vi "GOOP_ClassSettingsMemory.vi"(0 "Library Refnum":refnum<vi>, 1 "Action":T3, 2 "LvClassIconSettingsIn":T2 {"Frame thickness" min=1 max=3 step=1}, 3 "ItemIconIn":string, 5 "error in":errorcluster) -> (14 "Library Refnum":refnum<vi>, 15 "Found":bool, 16 "LvClassIconSettings":T2 {"Frame thickness" min=1 max=3 step=1}, 17 "ItemIcon":string, 18 "Type":T1, 19 "error out":errorcluster)   [LabVIEW 2020]
uses:
  <resource>/Framework/Providers/Open_GDS/ClassProviders/Common/LvClass_class/GDSLvClass_IconSettingsType.ctl
  <resource>/Framework/Providers/Open_GDS/SubVIs/GOOP_ClassSettingsMemory_Action.ctl
  <resource>/Framework/Providers/Open_GDS/ClassProviders/Common/LvIcon_class/GDSLvIcon_Type.ctl
  <resource>/Framework/Providers/Open_GDS/ClassProviders/Common/LvClass_class/GDSLvClass_IconSettingsNames.ctl
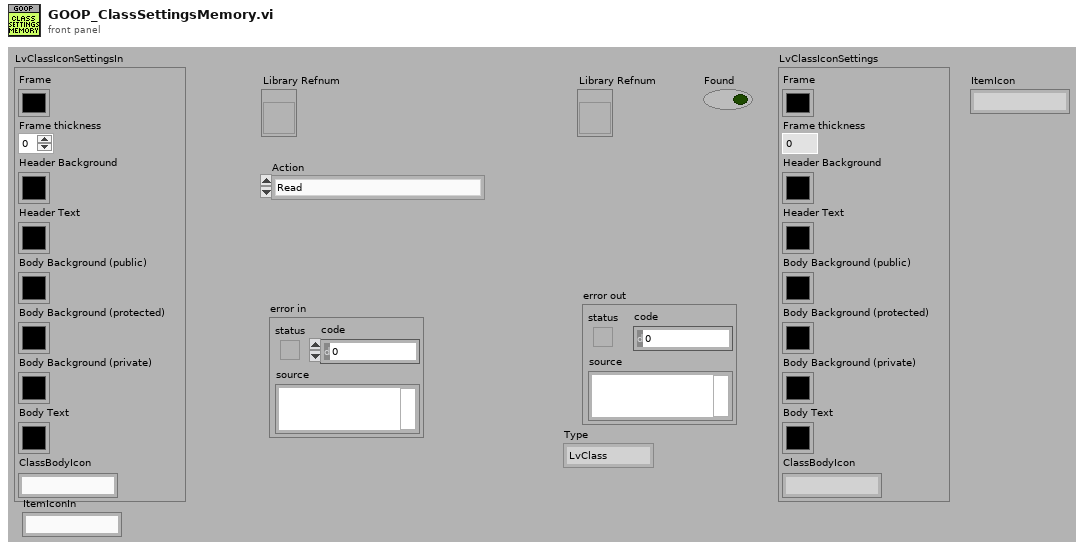
[diagram p1: front panel]
types:
  T1 = typedef "GDSLvIcon_Type.ctl" = enum16{"LvClass", "Library", "X-Control", "LvInterface"}
  T2 = typedef "GDSLvClass_IconSettingsType.ctl" = cluster{"Frame":u32, "Frame thickness":u8, "Header Background":u32, "Header Text":u32, "ColorPublic":u32, "ColorProtected":u32, "ColorPrivate":u32, "Body Text":u32, "ClassBodyIcon":string}
  T3 = typedef "GOOP_ClassSettingsMemory_Action.ctl" = enum16{"Read", "Write", "Read (ClassItemIconOnly)"}
  T4 = typedef "GDSLvClass_IconSettingsNames.ctl" = enum16{"EndevoGOOP_ColorFrame", "EndevoGOOP_FrameThickness", "EndevoGOOP_ColorHeader", "EndevoGOOP_ColorTextHeader", "EndevoGOOP_ColorPublic", "EndevoGOOP_ColorProtected", "EndevoGOOP_ColorPrivate", "EndevoGOOP_ColorTextBody", "EndevoGOOP_ClassItemIcon", "EndevoGOOP_ClassBodyIcon"}
  T5 = cluster{"LvClassIconSettingsIn":T2, "ItemIconIn":string}
  T6 = cluster{"LvClassIconSettings":T2, "ItemIcon":string}
  T7 = cluster{"LvClassIconSettings":T2, "ItemIcon":string}[]
  T8 = cluster{"LvClassIconSettingsIn":T2, "ItemIconIn":string}[]
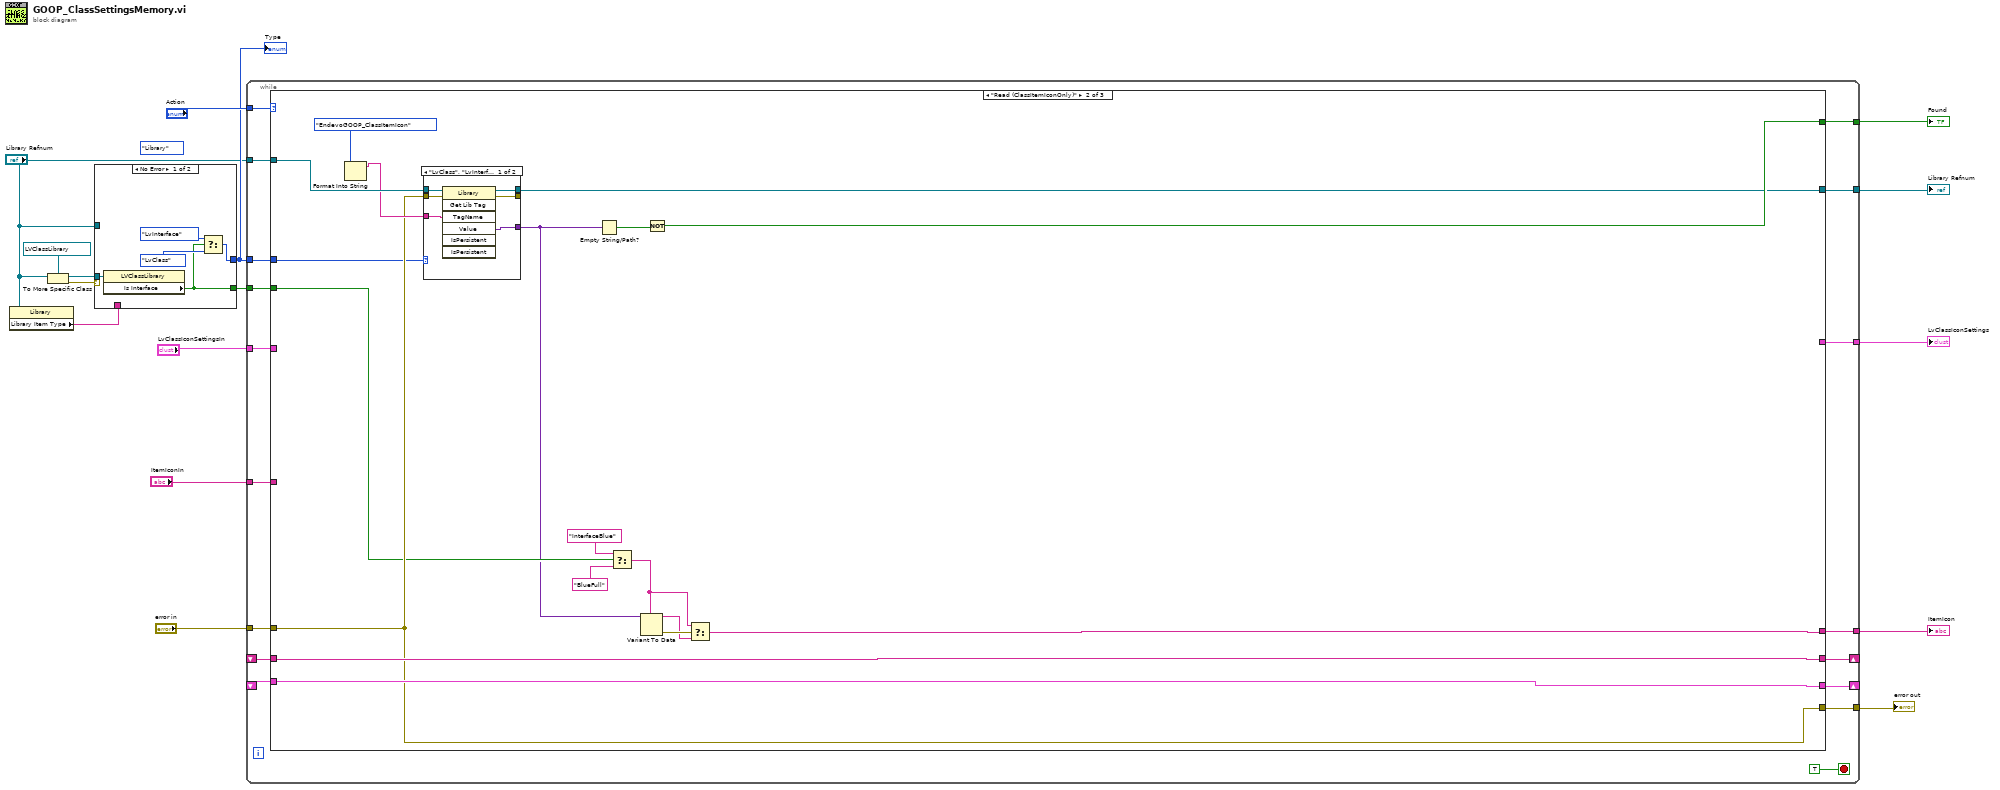
[diagram p0: block diagram]
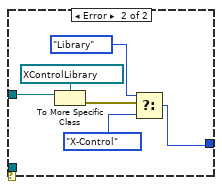
[diagram p2: hidden frame]
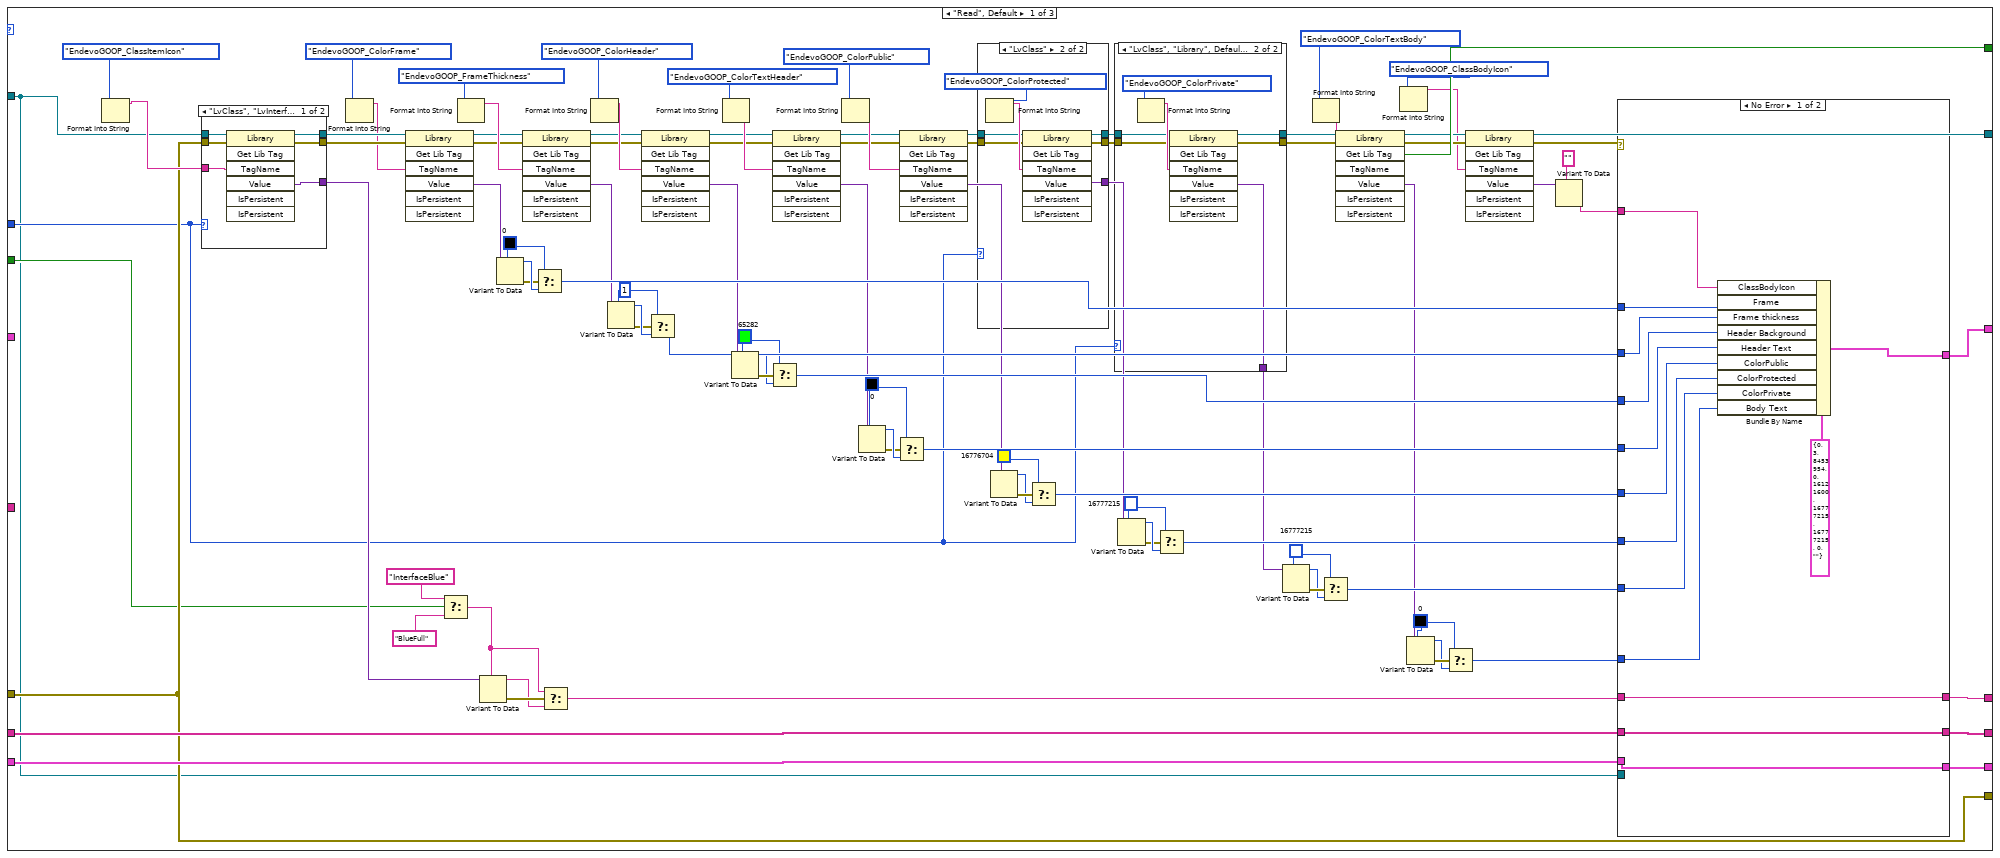
[diagram p3: hidden frame]
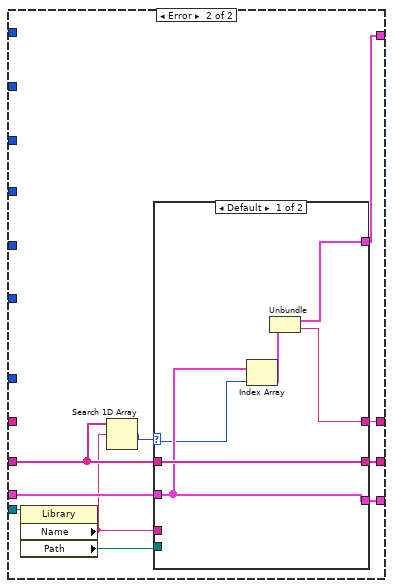
[diagram p7: hidden frame]
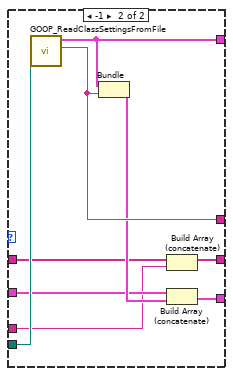
[diagram p8: hidden frame]
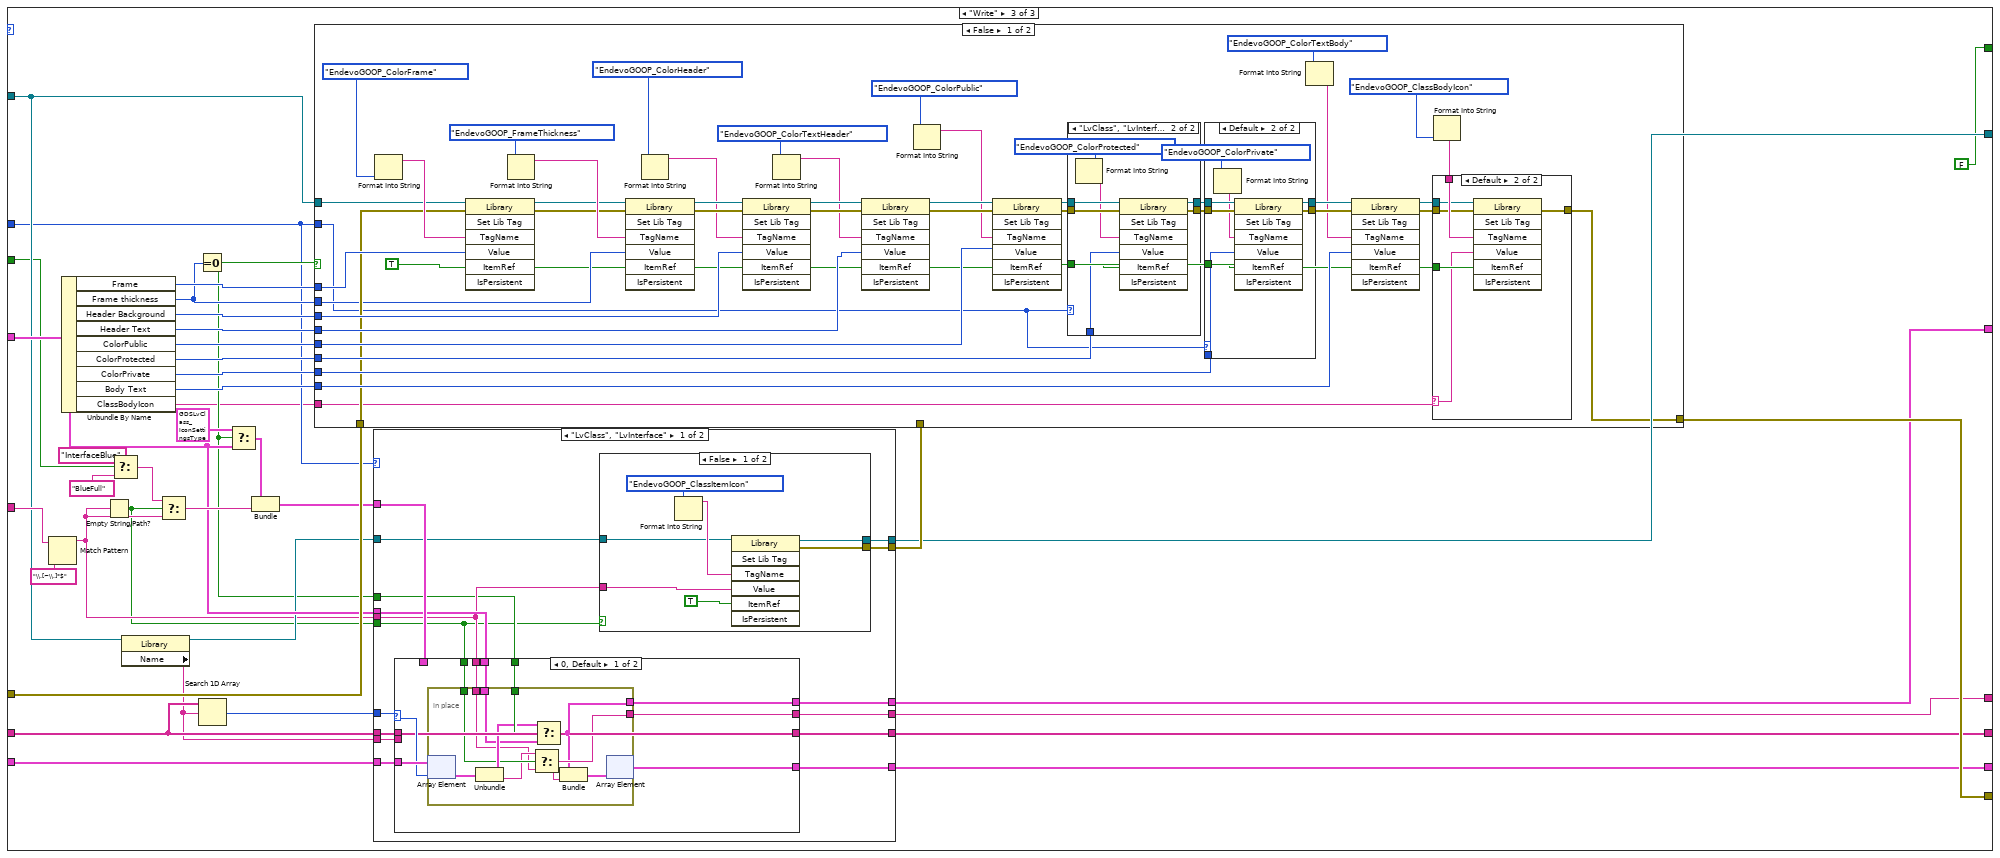
[diagram p10: hidden frame]
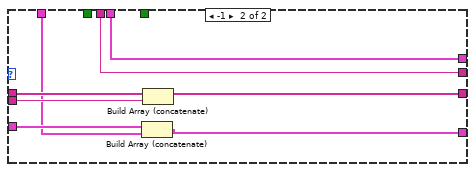
[diagram p12: hidden frame]
diagram:
  (unwired) GDSLvIcon_Type."Library" ("Type")
  n1 = property class="Library"(reference="Library Refnum") -> ("Library Item Type"=w3:string)  [unwired: 1 in, 2 out]
  n2 = To More Specific Class(target class=refnum<vi> refnum ("reference"), reference="Library Refnum") -> (specific class reference=w2:refnum<vi>, error out=w5:errorcluster)  [unwired: 1 in]
  n3 = case shown="No Error" w5 {
    tunnel: "Library Refnum" -> [_ w26]
    tunnel: [w18 w24] -> w6
    tunnel: w3 -> [_ _]
    tunnel: w2 -> [w21 _]
    tunnel: [w17 _] -> w1
    frame No Error {
      n4 = property class="LVClassLibrary"(reference=w21) -> ("Is Interface"=w17:bool)  [unwired: 1 in, 2 out]
      n5 = Select(t=GDSLvIcon_Type."LvInterface" ("Type"), s=w17, f=GDSLvIcon_Type."LvClass" ("Type")) -> (s? t:f=w18:T1)
    }
    frame Error {
      n6 = To More Specific Class(target class=refnum<vi> refnum ("reference"), reference=w26) -> (error out=w25:errorcluster)  [unwired: 1 in, 1 out]
      n7 = Select(t=GDSLvIcon_Type."Library" ("Type"), s=w25, f=GDSLvIcon_Type."X-Control" ("Type")) -> (s? t:f=w24:T1)
    }
  }
  "Type" <- w6
  n8 = while {
    tunnel: [w44] -> w16
    tunnel: [w43] -> w15
    tunnel: "Library Refnum" -> [w42]
    tunnel: "error in" -> [w41]
    tunnel: [w40] -> w13
    tunnel: [w39] -> w12
    shift-right: [w36] -> _
    shift-left: _ -> [w37]
    shift-right: [w35] -> _
    shift-left: _ -> [w34]
    tunnel: "Action" -> [w33]
    tunnel: "LvClassIconSettingsIn" -> [w32]
    tunnel: [w31] -> w9
    tunnel: "ItemIconIn" -> [w30]
    tunnel: w6 -> [w29]
    tunnel: w1 -> [w28]
    stop <- TRUE stop-if-true
    n9 = case shown="\"Read (ClassItemIconOnly)\"" w33 {
      tunnel: [w141 w224 w249] -> w44
      tunnel: [w140 _ w250] -> w43
      tunnel: w42 -> [w45 w222 w239]
      tunnel: w41 -> [w60 w216 w264]
      tunnel: [w101 w208 FALSE ("GetTag")] -> w40
      tunnel: [w55 w207 w242] -> w39
      tunnel: w37 -> [w64 w218 w261]
      tunnel: [w63 w218 w251] -> w36
      tunnel: [w62 w217 w252] -> w35
      tunnel: w34 -> [w61 w217 w255]
      tunnel: w32 -> [_ _ w253]
      tunnel: [w60 w216 w259] -> w31
      tunnel: w30 -> [_ _ w246]
      tunnel: w29 -> [w59 w215 w238]
      tunnel: w28 -> [w49 w214 w236]
      frame "Read", Default {
        w106 = u32 16777215 ("Frame")
        w97 = u32 0 ("Frame")
        w95 = u32 16777215 ("Frame")
        w89 = u32 16776704 ("Frame")
        w87 = u32 0 ("Frame")
        w81 = u32 65282 ("Frame")
        w79 = u8 1 ("Frame thickness")
        w77 = u32 0 ("Frame")
        n10 = Format Into String(GDSLvClass_IconSettingsNames."EndevoGOOP_ClassItemIcon" ("Enum")) -> (resulting string=w127:string)  [unwired: 3 in, 1 out]
        n11 = case shown="\"LvClass\", \"LvInterface\"" w59 {
          tunnel: [w165 _] -> w129
          tunnel: w45 -> [w164 w167]
          tunnel: w127 -> [w163 _]
          tunnel: [w162 w166] -> w126
          tunnel: [w161 w167] -> w125
          tunnel: w60 -> [w160 w166]
          frame "LvClass", "LvInterface" {
            n12 = invoke class="Library" method="Get Lib Tag"(reference=w164, error in=w160, "TagName"=w163) -> (reference out=w161:refnum<vi>, error out=w162:errorcluster, "Value"=w165:variant)  [unwired: 4 in, 4 out]
          }
          frame Default {
          }
        }
        n13 = Format Into String(GDSLvClass_IconSettingsNames."EndevoGOOP_ColorFrame" ("Enum")) -> (resulting string=w111:string)  [unwired: 3 in, 1 out]
        n14 = invoke class="Library" method="Get Lib Tag"(reference=w125, error in=w126, "TagName"=w111) -> (reference out=w65:refnum<vi>, error out=w112:errorcluster, "Value"=w71:variant)  [unwired: 4 in, 4 out]
        n15 = Select(t="InterfaceBlue", s=w49, f="BlueFull") -> (s? t:f=w46:string)
        n16 = Format Into String(GDSLvClass_IconSettingsNames."EndevoGOOP_FrameThickness" ("Enum")) -> (resulting string=w113:string)  [unwired: 3 in, 1 out]
        n17 = Variant To Data(type=w46, Variant=w129) -> (data=w128:string, error out=w130:errorcluster)  [unwired: 1 in]
        n18 = Variant To Data(type=w77, Variant=w71) -> (data=w76:u32, error out=w75:errorcluster)  [unwired: 1 in]
        n19 = invoke class="Library" method="Get Lib Tag"(reference=w65, error in=w112, "TagName"=w113) -> (reference out=w68:refnum<vi>, error out=w114:errorcluster, "Value"=w72:variant)  [unwired: 4 in, 4 out]
        n20 = Select(t=w77, s=w75, f=w76) -> (s? t:f=w131:u32)
        n21 = Select(t=w46, s=w130, f=w128) -> (s? t:f=w139:string)
        n22 = Format Into String(GDSLvClass_IconSettingsNames."EndevoGOOP_ColorHeader" ("Enum")) -> (resulting string=w115:string)  [unwired: 3 in, 1 out]
        n23 = Variant To Data(type=w79, Variant=w72) -> (data=w80:u8, error out=w78:errorcluster)  [unwired: 1 in]
        n24 = invoke class="Library" method="Get Lib Tag"(reference=w68, error in=w114, "TagName"=w115) -> (reference out=w66:refnum<vi>, error out=w67:errorcluster, "Value"=w84:variant)  [unwired: 4 in, 4 out]
        n25 = Select(t=w79, s=w78, f=w80) -> (s? t:f=w132:u8)
        n26 = Format Into String(GDSLvClass_IconSettingsNames."EndevoGOOP_ColorTextHeader" ("Enum")) -> (resulting string=w116:string)  [unwired: 3 in, 1 out]
        n27 = Variant To Data(type=w81, Variant=w84) -> (data=w82:u32, error out=w83:errorcluster)  [unwired: 1 in]
        n28 = Select(t=w81, s=w83, f=w82) -> (s? t:f=w133:u32)
        n29 = invoke class="Library" method="Get Lib Tag"(reference=w66, error in=w67, "TagName"=w116) -> (reference out=w69:refnum<vi>, error out=w70:errorcluster, "Value"=w88:variant)  [unwired: 4 in, 4 out]
        n30 = Format Into String(GDSLvClass_IconSettingsNames."EndevoGOOP_ColorPublic" ("Enum")) -> (resulting string=w117:string)  [unwired: 3 in, 1 out]
        n31 = Variant To Data(type=w87, Variant=w88) -> (data=w86:u32, error out=w85:errorcluster)  [unwired: 1 in]
        n32 = Select(t=w87, s=w85, f=w86) -> (s? t:f=w134:u32)
        n33 = invoke class="Library" method="Get Lib Tag"(reference=w69, error in=w70, "TagName"=w117) -> (reference out=w73:refnum<vi>, error out=w74:errorcluster, "Value"=w92:variant)  [unwired: 4 in, 4 out]
        n34 = case shown="\"LvClass\"" w59 {
          tunnel: [w142 w148] -> w103
          tunnel: [w143 w147] -> w102
          tunnel: [_ w146] -> w96
          tunnel: w74 -> [w142 w145]
          tunnel: w73 -> [w143 w144]
          frame Default {
          }
          frame "LvClass" {
            n35 = Format Into String(GDSLvClass_IconSettingsNames."EndevoGOOP_ColorProtected" ("Enum")) -> (resulting string=w149:string)  [unwired: 3 in, 1 out]
            n36 = invoke class="Library" method="Get Lib Tag"(reference=w144, error in=w145, "TagName"=w149) -> (reference out=w147:refnum<vi>, error out=w148:errorcluster, "Value"=w146:variant)  [unwired: 4 in, 4 out]
          }
        }
        n37 = Variant To Data(type=w89, Variant=w92) -> (data=w90:u32, error out=w91:errorcluster)  [unwired: 1 in]
        n38 = Select(t=w89, s=w91, f=w90) -> (s? t:f=w135:u32)
        n39 = case shown="\"LvClass\", \"Library\", Default" w59 {
          tunnel: [_ w157] -> w109
          tunnel: [w151 w156] -> w105
          tunnel: [w152 w155] -> w104
          tunnel: w103 -> [w151 w154]
          tunnel: w102 -> [w152 w153]
          frame "X-Control" {
          }
          frame "LvClass", "Library", Default {
            n40 = Format Into String(GDSLvClass_IconSettingsNames."EndevoGOOP_ColorPrivate" ("Enum")) -> (resulting string=w158:string)  [unwired: 3 in, 1 out]
            n41 = invoke class="Library" method="Get Lib Tag"(reference=w153, error in=w154, "TagName"=w158) -> (reference out=w155:refnum<vi>, error out=w156:errorcluster, "Value"=w157:variant)  [unwired: 4 in, 4 out]
          }
        }
        n42 = Variant To Data(type=w95, Variant=w96) -> (data=w94:u32, error out=w93:errorcluster)  [unwired: 1 in]
        n43 = Select(t=w95, s=w93, f=w94) -> (s? t:f=w136:u32)
        n44 = Variant To Data(type=w106, Variant=w109) -> (data=w107:u32, error out=w108:errorcluster)  [unwired: 1 in]
        n45 = Format Into String(GDSLvClass_IconSettingsNames."EndevoGOOP_ColorTextBody" ("Enum")) -> (resulting string=w118:string)  [unwired: 3 in, 1 out]
        n46 = Select(t=w106, s=w108, f=w107) -> (s? t:f=w137:u32)
        n47 = invoke class="Library" method="Get Lib Tag"(reference=w104, error in=w105, "TagName"=w118) -> (reference out=w58:refnum<vi>, error out=w57:errorcluster, "GetTag"=w101:bool, "Value"=w100:variant)  [unwired: 4 in, 3 out]
        n48 = Format Into String(GDSLvClass_IconSettingsNames."EndevoGOOP_ClassBodyIcon" ("Enum")) -> (resulting string=w53:string)  [unwired: 3 in, 1 out]
        n49 = Variant To Data(type=w97, Variant=w100) -> (data=w98:u32, error out=w99:errorcluster)  [unwired: 1 in]
        n50 = Select(t=w97, s=w99, f=w98) -> (s? t:f=w138:u32)
        n51 = invoke class="Library" method="Get Lib Tag"(reference=w58, error in=w57, "TagName"=w53) -> (reference out=w55:refnum<vi>, error out=w56:errorcluster, "Value"=w52:variant)  [unwired: 4 in, 4 out]
        n52 = Variant To Data(type="", Variant=w52) -> (data=w50:string)  [unwired: 1 in, 1 out]
        n53 = case shown="No Error" w56 {
          tunnel: w131 -> [w181 _]
          tunnel: w132 -> [w180 _]
          tunnel: w133 -> [w179 _]
          tunnel: w134 -> [w178 _]
          tunnel: w135 -> [w177 _]
          tunnel: w136 -> [w176 _]
          tunnel: w137 -> [w175 _]
          tunnel: w138 -> [w174 _]
          tunnel: w139 -> [w171 _]
          tunnel: [w172 w191] -> w140
          tunnel: [w171 w190] -> w141
          tunnel: w64 -> [w170 w186]
          tunnel: [w170 w189] -> w63
          tunnel: [w169 w188] -> w62
          tunnel: w61 -> [w169 w187]
          tunnel: w50 -> [w168 _]
          tunnel: w45 -> [_ w184]
          frame No Error {
            n54 = Bundle By Name(cluster=T2 {"Frame"=0, "Frame thickness"=3, "Header Background"=8453954, "Header Text"=0, "ColorPublic"=16121600, "ColorProtected"=16777215, "ColorPrivate"=16777215, "Body Text"=0, "ClassBodyIcon"=""} ("LvClassIconSettings"), "ClassBodyIcon"=w168, "Frame"=w181, "Frame thickness"=w180, "Header Background"=w179, "Header Text"=w178, "ColorPublic"=w177, "ColorProtected"=w176, "ColorPrivate"=w175, "Body Text"=w174) -> (w172:T2)
          }
          frame Error {
            n55 = property class="Library"(reference=w184) -> ("Name"=w183:string, "Path"=w182:path)  [unwired: 1 in, 2 out]
            n56 = Search 1D Array(1D array=w186, element=w183) -> (index of element=w185:i32)  [unwired: 1 in]
            n57 = case shown="Default" w185 {
              selector: w185 -> [w195 _]
              tunnel: w182 -> [_ w206]
              tunnel: [w193 w205] -> w191
              tunnel: [w192 w204] -> w190
              tunnel: [w197 w203] -> w189
              tunnel: [w196 w202] -> w188
              tunnel: w187 -> [w196 w200]
              tunnel: w186 -> [w197 w199]
              tunnel: w183 -> [_ w198]
              frame Default {
                n58 = Index Array(array=w196, index=w195) -> (element=w194:T5)
                n59 = Unbundle(w194) -> ("LvClassIconSettingsIn"=w193:T2, "ItemIconIn"=w192:string)
              }
              frame -1 {
                n60 = call <resource>:"GOOP_ReadClassSettingsFromFile.vi"("LvClassPath"=w206) -> ("ItemIcon"=w204:string, "LvClassIconSettings"=w205:T2)  [unwired: 8 in, 1 out]
                n61 = Bundle("LvClassIconSettings"=w205, "ItemIcon"=w204) -> (w201:T6)  [unwired: 1 in]
                n62 = Build Array (concatenate)(w199, w198) -> (w203:string[])
                n63 = Build Array (concatenate)(w200, w201) -> (w202:T7)
              }
            }
          }
        }
      }
      frame "Read (ClassItemIconOnly)" {
        n64 = Format Into String(GDSLvClass_IconSettingsNames."EndevoGOOP_ClassItemIcon" ("Enum")) -> (resulting string=w220:string)  [unwired: 3 in, 1 out]
        n65 = case shown="\"LvClass\", \"LvInterface\"" w215 {
          tunnel: [w230 _] -> w210
          tunnel: w222 -> [w229 w232]
          tunnel: w220 -> [w228 _]
          tunnel: [w227 w231] -> _
          tunnel: [w226 w232] -> w207
          tunnel: w216 -> [w225 w231]
          frame "LvClass", "LvInterface" {
            n66 = invoke class="Library" method="Get Lib Tag"(reference=w229, error in=w225, "TagName"=w228) -> (reference out=w226:refnum<vi>, error out=w227:errorcluster, "Value"=w230:variant)  [unwired: 4 in, 4 out]
          }
          frame Default {
          }
        }
        n67 = Empty String/Path?(string/path=w210) -> (empty?=w209:bool)
        n68 = Select(t="InterfaceBlue", s=w214, f="BlueFull") -> (s? t:f=w211:string)
        n69 = Variant To Data(type=w211, Variant=w210) -> (data=w221:string, error out=w223:errorcluster)  [unwired: 1 in]
        n70 = Not(x=w209) -> (.not. x?=w208:bool)
        n71 = Select(t=w211, s=w223, f=w221) -> (s? t:f=w224:string)
      }
      frame "Write" {
        n72 = Match Pattern(string=w246, regular expression="\\.[~\\.]*$") -> (before substring=w245:string)  [unwired: 1 in, 3 out]
        n73 = Unbundle By Name(w253) -> ("Frame"=w270:u32, "Frame thickness"=w263:u8, "Header Background"=w271:u32, "Header Text"=w269:u32, "ColorPublic"=w268:u32, "ColorProtected"=w267:u32, "ColorPrivate"=w266:u32, "Body Text"=w265:u32, "ClassBodyIcon"=w237:string)
        n74 = Empty String/Path?(string/path=w245) -> (empty?=w240:bool)
        n75 = Select(t="InterfaceBlue", s=w236, f="BlueFull") -> (s? t:f=w234:string)
        n76 = property class="Library"(reference=w239) -> (reference out=w248:refnum<vi>, "Name"=w260:string)  [unwired: 1 in, 1 out]
        n77 = Select(t=w234, s=w240, f=w245) -> (s? t:f=w258:string)
        n78 = Equal To 0?(x=w263) -> (x = 0?=w244:bool)
        n79 = Search 1D Array(1D array=w261, element=w260) -> (index of element=w262:i32)  [unwired: 1 in]
        n80 = Select(t=T2 {"Frame"=0, "Frame thickness"=3, "Header Background"=8453954, "Header Text"=0, "ColorPublic"=16121600, "ColorProtected"=16777215, "ColorPrivate"=16777215, "Body Text"=0, "ClassBodyIcon"=""} ("LvClassIconSettings"), s=w244, f=w253) -> (s? t:f=w256:T2)
        n81 = Bundle("LvClassIconSettingsIn"=w256, "ItemIconIn"=w258) -> (w254:T5)  [unwired: 1 in]
        n82 = case shown="\"LvClass\", \"LvInterface\"" w238 {
          tunnel: w262 -> [w287 _]
          tunnel: w261 -> [w286 w326]
          tunnel: w260 -> [w285 _]
          tunnel: w255 -> [w284 w327]
          tunnel: w254 -> [w283 _]
          tunnel: w253 -> [w282 w324]
          tunnel: [w281 w327] -> w252
          tunnel: [w280 w326] -> w251
          tunnel: [w279 w324] -> w250
          tunnel: [w278 w325] -> w249
          tunnel: w248 -> [w277 w328]
          tunnel: w245 -> [w276 w325]
          tunnel: w244 -> [w275 _]
          tunnel: [w274 _] -> w243
          tunnel: [w273 w328] -> w242
          tunnel: w240 -> [w272 _]
          frame "LvClass", "LvInterface" {
            n83 = case shown="0, Default" w287 {
              selector: w287 -> [w304 _]
              tunnel: w286 -> [w297 w323]
              tunnel: w285 -> [_ w322]
              tunnel: w284 -> [w305 w321]
              tunnel: w283 -> [_ w320]
              tunnel: w275 -> [w303 _]
              tunnel: w282 -> [w302 w317]
              tunnel: w272 -> [w301 _]
              tunnel: w276 -> [w300 w316]
              tunnel: [w296 w319] -> w281
              tunnel: [w297 w318] -> w280
              tunnel: [w299 w316] -> w278
              tunnel: [w298 w317] -> w279
              frame 0, Default {
                n84 = in-place {
                  in-place-border: w303 -> [w313]
                  in-place-border: w302 -> [w311]
                  in-place-border: w301 -> [w310]
                  in-place-border: w300 -> [w308]
                  in-place-border: [w307] -> w299
                  in-place-border: [w306] -> w298
                  n85 = in-place-array #1(w305, w304) -> (w315:T5)
                  n86 = Unbundle(w315) -> ("LvClassIconSettingsIn"=w312:T2, "ItemIconIn"=w309:string)
                  n87 = Select(t=w309, s=w310, f=w308) -> (s? t:f=w307:string)
                  n88 = Select(t=w312, s=w313, f=w311) -> (s? t:f=w306:T2)
                  n89 = Bundle("LvClassIconSettingsIn"=w306, "ItemIconIn"=w307) -> (w314:T5)  [unwired: 1 in]
                  n90 = in-place-array #1(w314) -> (w296:T8)  [unwired: 1 out]
                }
              }
              frame -1 {
                n91 = Build Array (concatenate)(w321, w320) -> (w319:T8)
                n92 = Build Array (concatenate)(w323, w322) -> (w318:string[])
              }
            }
            n93 = case shown="False" w272 {
              tunnel: w277 -> [w291 w295]
              tunnel: w276 -> [w290 _]
              tunnel: [w289 _] -> w274
              tunnel: [w288 w295] -> w273
              frame False {
                n94 = Format Into String(GDSLvClass_IconSettingsNames."EndevoGOOP_ClassItemIcon" ("Enum")) -> (resulting string=w293:string)  [unwired: 3 in, 1 out]
                n95 = invoke class="Library" method="Set Lib Tag"(reference=w291, "TagName"=w293, "Value"=w290, "ItemRef"=TRUE ("Is Persistent")) -> (reference out=w288:refnum<vi>, error out=w289:errorcluster)  [unwired: 3 in, 5 out]
              }
              frame True {
              }
            }
          }
          frame "Library", "X-Control", Default {
            # "This is a Library or a XControl, this should only be done for classes"
          }
        }
        n96 = case shown="False" w244 {
          tunnel: w271 -> [w347 _]
          tunnel: w270 -> [w346 _]
          tunnel: w269 -> [w345 _]
          tunnel: w268 -> [w344 _]
          tunnel: w267 -> [w343 _]
          tunnel: w266 -> [w342 _]
          tunnel: w265 -> [w341 _]
          tunnel: w239 -> [w340 _]
          tunnel: w264 -> [w339 w400]
          tunnel: w263 -> [w337 _]
          tunnel: [w332 w400] -> w259
          tunnel: w243 -> [_ _]
          tunnel: w238 -> [w336 _]
          tunnel: w237 -> [w329 _]
          frame False {
            w330 = TRUE ("Is Persistent")
            n97 = Format Into String(GDSLvClass_IconSettingsNames."EndevoGOOP_ColorFrame" ("Enum")) -> (resulting string=w348:string)  [unwired: 3 in, 1 out]
            n98 = invoke class="Library" method="Set Lib Tag"(reference=w340, error in=w339, "TagName"=w348, "Value"=w346, "ItemRef"=w330) -> (reference out=w350:refnum<vi>, error out=w349:errorcluster)  [unwired: 2 in, 5 out]
            n99 = Format Into String(GDSLvClass_IconSettingsNames."EndevoGOOP_FrameThickness" ("Enum")) -> (resulting string=w351:string)  [unwired: 3 in, 1 out]
            n100 = invoke class="Library" method="Set Lib Tag"(reference=w350, error in=w349, "TagName"=w351, "Value"=w337, "ItemRef"=w330) -> (reference out=w372:refnum<vi>, error out=w371:errorcluster)  [unwired: 2 in, 5 out]
            n101 = Format Into String(GDSLvClass_IconSettingsNames."EndevoGOOP_ColorHeader" ("Enum")) -> (resulting string=w352:string)  [unwired: 3 in, 1 out]
            n102 = invoke class="Library" method="Set Lib Tag"(reference=w372, error in=w371, "TagName"=w352, "Value"=w347, "ItemRef"=w330) -> (reference out=w368:refnum<vi>, error out=w367:errorcluster)  [unwired: 2 in, 5 out]
            n103 = Format Into String(GDSLvClass_IconSettingsNames."EndevoGOOP_ColorTextHeader" ("Enum")) -> (resulting string=w353:string)  [unwired: 3 in, 1 out]
            n104 = invoke class="Library" method="Set Lib Tag"(reference=w368, error in=w367, "TagName"=w353, "Value"=w345, "ItemRef"=w330) -> (reference out=w370:refnum<vi>, error out=w369:errorcluster)  [unwired: 2 in, 5 out]
            n105 = Format Into String(GDSLvClass_IconSettingsNames."EndevoGOOP_ColorPublic" ("Enum")) -> (resulting string=w354:string)  [unwired: 3 in, 1 out]
            n106 = invoke class="Library" method="Set Lib Tag"(reference=w370, error in=w369, "TagName"=w354, "Value"=w344, "ItemRef"=w330) -> (reference out=w366:refnum<vi>, error out=w365:errorcluster)  [unwired: 2 in, 5 out]
            n107 = case shown="\"LvClass\", \"LvInterface\"" w336 {
              tunnel: w366 -> [w391 w399]
              tunnel: w365 -> [w390 w398]
              tunnel: [w391 w397] -> w364
              tunnel: [w390 w396] -> w363
              tunnel: w343 -> [_ w393]
              tunnel: w330 -> [_ w392]
              frame Default {
              }
              frame "LvClass", "LvInterface" {
                n108 = Format Into String(GDSLvClass_IconSettingsNames."EndevoGOOP_ColorProtected" ("Enum")) -> (resulting string=w394:string)  [unwired: 3 in, 1 out]
                n109 = invoke class="Library" method="Set Lib Tag"(reference=w399, error in=w398, "TagName"=w394, "Value"=w393, "ItemRef"=w392) -> (reference out=w397:refnum<vi>, error out=w396:errorcluster)  [unwired: 2 in, 5 out]
              }
            }
            n110 = case shown="Default" w336 {
              tunnel: w364 -> [w381 w389]
              tunnel: w363 -> [w380 w388]
              tunnel: [w381 w387] -> w362
              tunnel: [w380 w386] -> w361
              tunnel: w342 -> [_ w384]
              tunnel: w330 -> [_ w383]
              frame "X-Control" {
              }
              frame Default {
                n111 = Format Into String(GDSLvClass_IconSettingsNames."EndevoGOOP_ColorPrivate" ("Enum")) -> (resulting string=w385:string)  [unwired: 3 in, 1 out]
                n112 = invoke class="Library" method="Set Lib Tag"(reference=w389, error in=w388, "TagName"=w385, "Value"=w384, "ItemRef"=w383) -> (reference out=w387:refnum<vi>, error out=w386:errorcluster)  [unwired: 2 in, 5 out]
              }
            }
            n113 = Format Into String(GDSLvClass_IconSettingsNames."EndevoGOOP_ColorTextBody" ("Enum")) -> (resulting string=w355:string)  [unwired: 3 in, 1 out]
            n114 = invoke class="Library" method="Set Lib Tag"(reference=w362, error in=w361, "TagName"=w355, "Value"=w341, "ItemRef"=w330) -> (reference out=w333:refnum<vi>, error out=w334:errorcluster)  [unwired: 2 in, 5 out]
            n115 = Format Into String(GDSLvClass_IconSettingsNames."EndevoGOOP_ClassBodyIcon" ("Enum")) -> (resulting string=w335:string)  [unwired: 3 in, 1 out]
            n116 = case shown="Default" w329 {
              selector: w329 -> [_ w374]
              tunnel: w335 -> [_ w379]
              tunnel: w334 -> [w373 w378]
              tunnel: w333 -> [_ w377]
              tunnel: [w373 w376] -> w332
              tunnel: w330 -> [_ w375]
              frame "" {
              }
              frame Default {
                n117 = invoke class="Library" method="Set Lib Tag"(reference=w377, error in=w378, "TagName"=w379, "Value"=w374, "ItemRef"=w375) -> (error out=w376:errorcluster)  [unwired: 2 in, 6 out]
              }
            }
          }
          frame True {
          }
        }
      }
    }
  }
  "ItemIcon" <- w16
  "LvClassIconSettings" <- w15
  "Found" <- w13
  "Library Refnum" <- w12
  "error out" <- w9
